vi "Spartan HTTP Connection Server.vi"(4 "error in (no error)":errorcluster, 6 "Handlers to Init (4)":i32=4, 7 "function (init)":enum16{"init", "finish"}(ring)) -> (0 "error out":errorcluster)   [LabVIEW 2011]
uses:
  Spartan HTTP Server Globals.vi
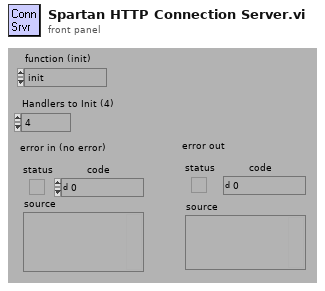
[diagram p1: front panel]
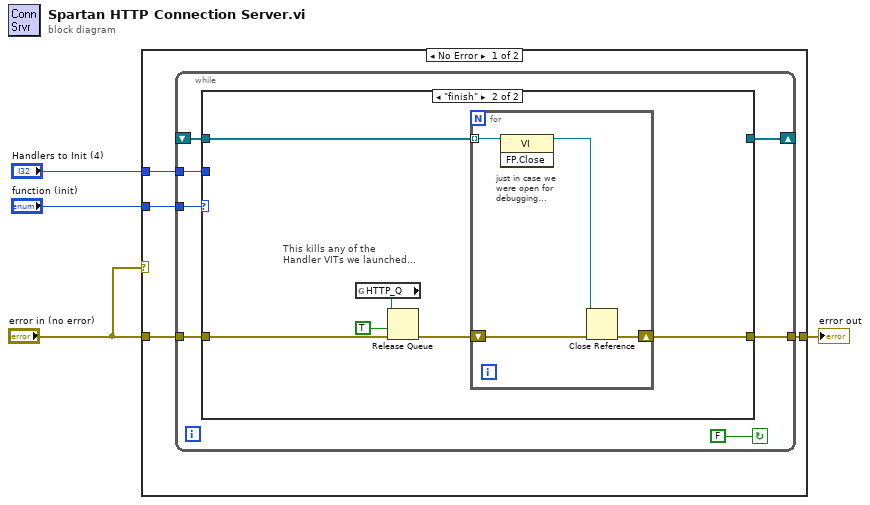
[diagram p0: block diagram]
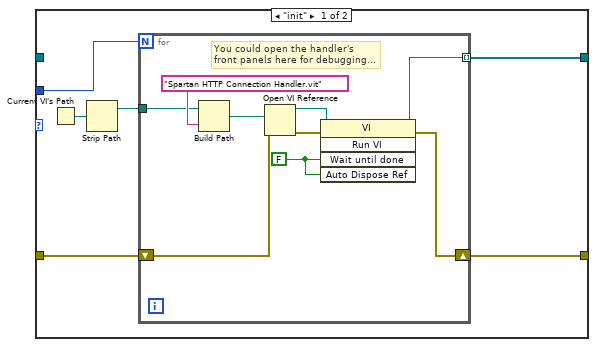
[diagram p2: hidden frame]
diagram:
  n1 = case shown="No Error" "error in (no error)" {
    tunnel: "Handlers to Init (4)" -> [w8 _]
    tunnel: "function (init)" -> [w7 _]
    tunnel: "error in (no error)" -> [w6 w41]
    tunnel: [w5 w41] -> w2
    frame No Error {
      n2 = while {
        shift-left: _ -> [w14]
        shift-right: [w15] -> _
        tunnel: w8 -> [w12]
        tunnel: w7 -> [w11]
        tunnel: w6 -> [w10]
        tunnel: [w9] -> w5
        stop <- FALSE continue-if-true
        n3 = case shown="\"finish\"" w11 {
          tunnel: [w18 _] -> w15
          tunnel: w14 -> [_ w36]
          tunnel: w12 -> [w19 _]
          tunnel: w10 -> [w17 w33]
          tunnel: [w16 w31] -> w9
          frame "init" {
            n4 = Current VI's Path() -> (path=w21:path)
            n5 = Strip Path(path=w21) -> (stripped path=w20:path)  [unwired: 1 out]
            n6 = for {
              N: w19 -> [_]
              tunnel: w20 -> [w25]
              tunnel: [w26] -> w18 mode=indexing
              shift-right: [w22] -> w16
              shift-left: w17 -> [w23]
              w27 = FALSE ("Wait until done")
              # "You could open the handler's\nfront panels here for debugging..."
              n7 = Build Path(base path=w25, name or relative path="Spartan HTTP Connection Handler.vit") -> (appended path=w30:path)
              n8 = Open VI Reference(vi path=w30, error in (no error)=w23) -> (vi reference=w24:refnum<vi>, error out=w29:errorcluster)  [unwired: 4 out]
              n9 = invoke class="VI" method="Run VI"(reference=w24, error in=w29, "Wait until done"=w27, "Auto Dispose Ref"=w27) -> (reference out=w26:refnum<vi>, error out=w22:errorcluster)  [unwired: 1 in, 3 out]
            }
          }
          frame "finish" {
            # "This kills any of the\nHandler VITs we launched..."
            n10 = global read "Spartan HTTP Server Globals.vi" "HTTP_Q"() -> (w34:refnum<queue>)
            n11 = Release Queue(queue=w34, force destroy? (F)=TRUE, error in (no error)=w33) -> (error out=w32:errorcluster)  [unwired: 2 out]
            n12 = for {
              tunnel: w36 -> [w40] mode=indexing
              shift-right: [w37] -> w31
              shift-left: w32 -> [w38]
              # "just in case we\nwere open for\ndebugging..."
              n13 = invoke class="VI" method="FP.Close"(reference=w40) -> (reference out=w39:refnum<vi>)  [unwired: 2 in, 2 out]
              n14 = Close Reference(reference=w39, error in (no error)=w38) -> (error out=w37:errorcluster)
            }
          }
        }
      }
    }
    frame Error {
      # "Bypass on ERROR"
    }
  }
  "error out" <- w2
